vi "Check Scan Error.vi"(8 "error in (no error)":errorcluster {"code" format="%x"}, 10 "Response Input":string, 11 "VISA resource name":refnum<visa-resource-name>) -> (0 "error out":errorcluster {"code" format="%x"}, 2 "Response Output":string, 3 "VISA resource name out":refnum<visa-resource-name>)   [LabVIEW 2023, in "Bronkhorst FLOW-BUS.lvlib"]
doc: "This VI checks if the response string after a write/read sequence contains a status message. If is does, the error or warning contained in the status message is output in the <b>error out</b> cluster. \n\nFor information about the structure of error messages, please refer to chapter 3.3.3 and 3.6 of document 9.17.027."
uses:
  Bronkhorst FLOW-BUS.lvlib
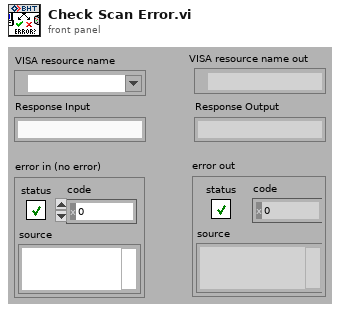
[diagram p1: front panel]
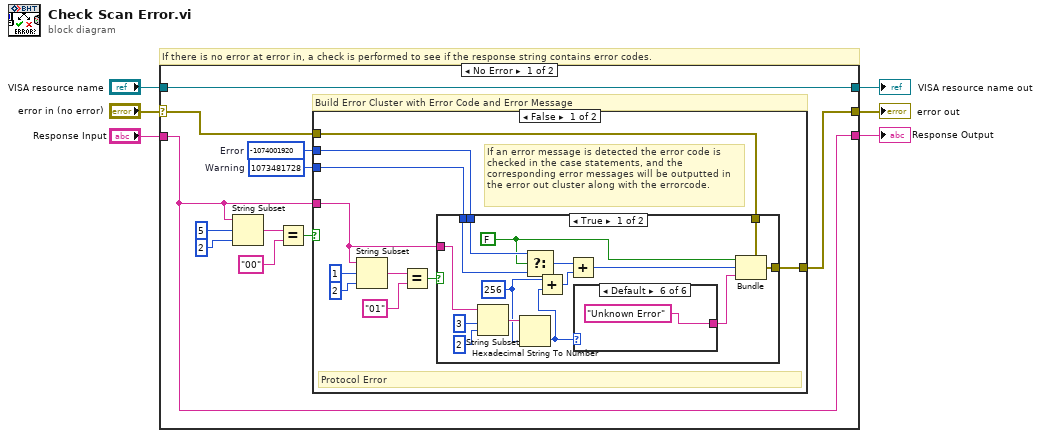
[diagram p0: block diagram]
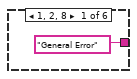
[diagram p2: hidden frame]
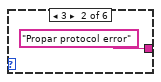
[diagram p3: hidden frame]
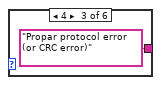
[diagram p4: hidden frame]
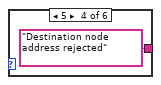
[diagram p5: hidden frame]
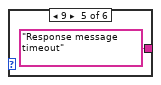
[diagram p6: hidden frame]
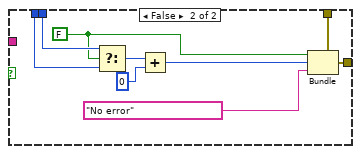
[diagram p7: hidden frame]
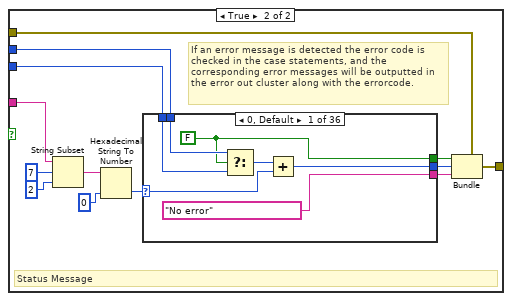
[diagram p8: hidden frame]
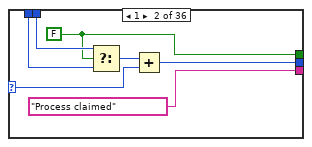
[diagram p9: hidden frame]
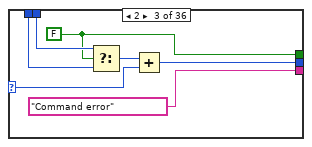
[diagram p10: hidden frame]
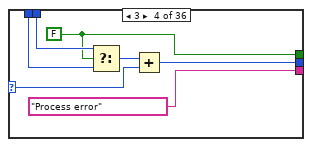
[diagram p11: hidden frame]
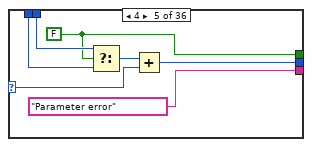
[diagram p12: hidden frame]
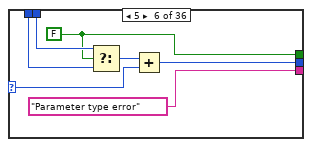
[diagram p13: hidden frame]
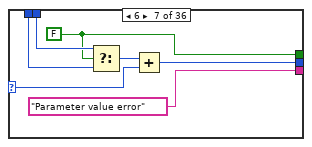
[diagram p14: hidden frame]
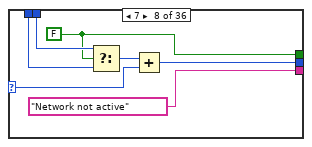
[diagram p15: hidden frame]
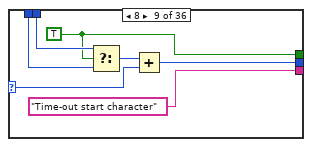
[diagram p16: hidden frame]
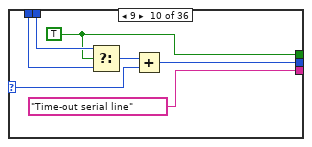
[diagram p17: hidden frame]
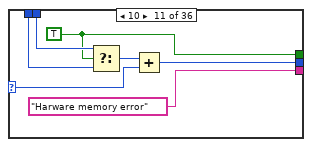
[diagram p18: hidden frame]
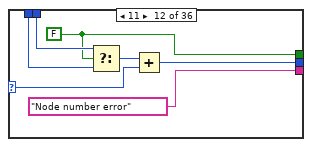
[diagram p19: hidden frame]
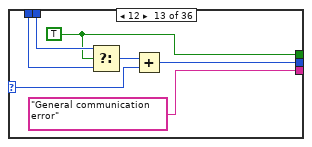
[diagram p20: hidden frame]
diagram:
  # "If there is no error at error in, a check is performed to see if the response string contains error codes."
  n1 = case shown="No Error" "error in (no error)" {
    selector: "error in (no error)" -> [w13 w325]
    tunnel: [w12 w325] -> w6
    tunnel: "Response Input" -> [w7 w323]
    tunnel: "VISA resource name" -> [w11 w324]
    tunnel: [w11 w324] -> w2
    tunnel: [w7 w323] -> w1
    frame No Error {
      w8 = 1073481728  # Warning
      w9 = -1074001920  # Error
      # "Build Error Cluster with Error Code and Error Message"
      n2 = String Subset(string=w7, offset (0)=u32 5 ("byte count (0)"), length (rest)=u32 2 ("byte count (0)")) -> (substring=w15:string)
      n3 = Equal?(x=w15, y="00" ("write buffer (\"\")")) -> (x = y?=w10:bool)
      n4 = case shown="False" w10 {
        tunnel: w7 -> [w20 w70]
        tunnel: w13 -> [w21 w66]
        tunnel: [w22 w65] -> w12
        tunnel: w9 -> [w19 w59]
        tunnel: w8 -> [w18 w58]
        frame False {
          # "Protocol Error"
          # "If an error message is detected the error code is checked in the case statements, and the corresponding error messages will be outputted in the error out cluster along with the errorcode."
          n5 = String Subset(string=w20, offset (0)=u32 1 ("byte count (0)"), length (rest)=u32 2 ("byte count (0)")) -> (substring=w23:string)
          n6 = Equal?(x=w23, y="01" ("write buffer (\"\")")) -> (x = y?=w26:bool)
          n7 = case shown="True" w26 {
            tunnel: w18 -> [w34 w55]
            tunnel: w19 -> [w35 w56]
            tunnel: w20 -> [w33 _]
            tunnel: [w32 w54] -> w22
            tunnel: w21 -> [w29 w52]
            frame True {
              w37 = 256 ("byte count (0)")
              w28 = FALSE
              n8 = String Subset(string=w33, offset (0)=u32 3 ("byte count (0)"), length (rest)=u32 2 ("byte count (0)")) -> (substring=w38:string)
              n9 = Hexadecimal String To Number(string=w38, default (0uL)=w37) -> (number=w36:i32)  [unwired: 1 in, 1 out]
              n10 = Select(t=w35, s=w28, f=w34) -> (s? t:f=w42:i32)
              n11 = Add(x=w37, y=w36) -> (x+y=w39:i32)
              n12 = Add(x=w42, y=w39) -> (x+y=w30:i32)
              n13 = case shown="Default" w36 {
                tunnel: ["General Error" "Propar protocol error" "Propar protocol error (or CRC error)" "Destination node address rejected" "Response message timeout" "Unknown Error"] -> w31
                frame 1, 2, 8 {
                }
                frame 3 {
                }
                frame 4 {
                }
                frame 5 {
                }
                frame 9 {
                }
                frame Default {
                }
              }
              n14 = Bundle(cluster=w29, "status"=w28, "code"=w30, "source"=w31) -> (w32:errorcluster)
            }
            frame False {
              w50 = FALSE
              n15 = Select(t=w56, s=w50, f=w55) -> (s? t:f=w57:i32)
              n16 = Add(x=w57, y=0) -> (x+y=w53:i32)
              n17 = Bundle(cluster=w52, "status"=w50, "code"=w53, "source"="No error") -> (w54:errorcluster)
            }
          }
        }
        frame True {
          # "Status Message"
          # "If an error message is detected the error code is checked in the case statements, and the corresponding error messages will be outputted in the error out cluster along with the errorcode."
          n18 = String Subset(string=w70, offset (0)=u32 7 ("byte count (0)"), length (rest)=u32 2 ("byte count (0)")) -> (substring=w67:string)
          n19 = Hexadecimal String To Number(string=w67, default (0uL)=0 ("I32")) -> (number=w63:i32)  [unwired: 1 in, 1 out]
          n20 = case shown="0, Default" w63 {
            selector: w63 -> [w73 w80 w87 w94 w101 w108 w115 w122 w129 w136 w143 w150 w157 w164 w171 w178 w185 w192 w199 w206 w213 w220 w227 w234 w241 w248 w255 w262 w269 w276 w283 w290 w297 w304 w311 w318]
            tunnel: w58 -> [w76 w83 w90 w97 w104 w111 w118 w125 w132 w139 w146 w153 w160 w167 w174 w181 w188 w195 w202 w209 w216 w223 w230 w237 w244 w251 w258 w265 w272 w279 w286 w293 w300 w307 w314 w321]
            tunnel: w59 -> [w75 w82 w89 w96 w103 w110 w117 w124 w131 w138 w145 w152 w159 w166 w173 w180 w187 w194 w201 w208 w215 w222 w229 w236 w243 w250 w257 w264 w271 w278 w285 w292 w299 w306 w313 w320]
            tunnel: [w74 w81 w88 w95 w102 w109 w116 w123 w130 w137 w144 w151 w158 w165 w172 w179 w186 w193 w200 w207 w214 w221 w228 w235 w242 w249 w256 w263 w270 w277 w284 w291 w298 w305 w312 w319] -> w60
            tunnel: ["No error" "Process claimed" "Command error" "Process error" "Parameter error" "Parameter type error" "Parameter value error" "Network not active" "Time-out start character" "Time-out serial line" "Harware memory error" "Node number error" "General communication error" "Read only parameter" "Error PC-communication" "No RS232 connection" "PC out of memory" "Write only parameter" "System configuration unknown" "No free node address" "Wrong interface type" "Error serial port connection" "Error opening communication" "Communication error" "Error interface bus master" "Timeout answer" "No start character" "Error first digit" "Buffer overflow in host" "Buffer overflow" "No answer found" "Error closing communication" "Synchronisation error" "Send error" "Protocol error" "Buffer overflow in module"] -> w62
            tunnel: [w71 w78 w85 w92 w99 w106 w113 w120 w127 w134 w141 w148 w155 w162 w169 w176 w183 w190 w197 w204 w211 w218 w225 w232 w239 w246 w253 w260 w267 w274 w281 w288 w295 w302 w309 w316] -> w61
            frame 0, Default {
              w74 = FALSE
              n21 = Select(t=w75, s=w74, f=w76) -> (s? t:f=w77:i32)
              n22 = Add(x=w77, y=w73) -> (x+y=w71:i32)
            }
            frame 1 {
              w81 = FALSE
              n23 = Select(t=w82, s=w81, f=w83) -> (s? t:f=w84:i32)
              n24 = Add(x=w84, y=w80) -> (x+y=w78:i32)
            }
            frame 2 {
              w88 = FALSE
              n25 = Select(t=w89, s=w88, f=w90) -> (s? t:f=w91:i32)
              n26 = Add(x=w91, y=w87) -> (x+y=w85:i32)
            }
            frame 3 {
              w95 = FALSE
              n27 = Select(t=w96, s=w95, f=w97) -> (s? t:f=w98:i32)
              n28 = Add(x=w98, y=w94) -> (x+y=w92:i32)
            }
            frame 4 {
              w102 = FALSE
              n29 = Select(t=w103, s=w102, f=w104) -> (s? t:f=w105:i32)
              n30 = Add(x=w105, y=w101) -> (x+y=w99:i32)
            }
            frame 5 {
              w109 = FALSE
              n31 = Select(t=w110, s=w109, f=w111) -> (s? t:f=w112:i32)
              n32 = Add(x=w112, y=w108) -> (x+y=w106:i32)
            }
            frame 6 {
              w116 = FALSE
              n33 = Select(t=w117, s=w116, f=w118) -> (s? t:f=w119:i32)
              n34 = Add(x=w119, y=w115) -> (x+y=w113:i32)
            }
            frame 7 {
              w123 = FALSE
              n35 = Select(t=w124, s=w123, f=w125) -> (s? t:f=w126:i32)
              n36 = Add(x=w126, y=w122) -> (x+y=w120:i32)
            }
            frame 8 {
              w130 = TRUE
              n37 = Select(t=w131, s=w130, f=w132) -> (s? t:f=w133:i32)
              n38 = Add(x=w133, y=w129) -> (x+y=w127:i32)
            }
            frame 9 {
              w137 = TRUE
              n39 = Select(t=w138, s=w137, f=w139) -> (s? t:f=w140:i32)
              n40 = Add(x=w140, y=w136) -> (x+y=w134:i32)
            }
            frame 10 {
              w144 = TRUE
              n41 = Select(t=w145, s=w144, f=w146) -> (s? t:f=w147:i32)
              n42 = Add(x=w147, y=w143) -> (x+y=w141:i32)
            }
            frame 11 {
              w151 = FALSE
              n43 = Select(t=w152, s=w151, f=w153) -> (s? t:f=w154:i32)
              n44 = Add(x=w154, y=w150) -> (x+y=w148:i32)
            }
            frame 12 {
              w158 = TRUE
              n45 = Select(t=w159, s=w158, f=w160) -> (s? t:f=w161:i32)
              n46 = Add(x=w161, y=w157) -> (x+y=w155:i32)
            }
            frame 13 {
              w165 = FALSE
              n47 = Select(t=w166, s=w165, f=w167) -> (s? t:f=w168:i32)
              n48 = Add(x=w168, y=w164) -> (x+y=w162:i32)
            }
            frame 14 {
              w172 = TRUE
              n49 = Select(t=w173, s=w172, f=w174) -> (s? t:f=w175:i32)
              n50 = Add(x=w175, y=w171) -> (x+y=w169:i32)
            }
            frame 15 {
              w179 = TRUE
              n51 = Select(t=w180, s=w179, f=w181) -> (s? t:f=w182:i32)
              n52 = Add(x=w182, y=w178) -> (x+y=w176:i32)
            }
            frame 16 {
              w186 = TRUE
              n53 = Select(t=w187, s=w186, f=w188) -> (s? t:f=w189:i32)
              n54 = Add(x=w189, y=w185) -> (x+y=w183:i32)
            }
            frame 17 {
              w193 = FALSE
              n55 = Select(t=w194, s=w193, f=w195) -> (s? t:f=w196:i32)
              n56 = Add(x=w196, y=w192) -> (x+y=w190:i32)
            }
            frame 18 {
              w200 = TRUE
              n57 = Select(t=w201, s=w200, f=w202) -> (s? t:f=w203:i32)
              n58 = Add(x=w203, y=w199) -> (x+y=w197:i32)
            }
            frame 19 {
              w207 = TRUE
              n59 = Select(t=w208, s=w207, f=w209) -> (s? t:f=w210:i32)
              n60 = Add(x=w210, y=w206) -> (x+y=w204:i32)
            }
            frame 20 {
              w214 = TRUE
              n61 = Select(t=w215, s=w214, f=w216) -> (s? t:f=w217:i32)
              n62 = Add(x=w217, y=w213) -> (x+y=w211:i32)
            }
            frame 21 {
              w221 = TRUE
              n63 = Select(t=w222, s=w221, f=w223) -> (s? t:f=w224:i32)
              n64 = Add(x=w224, y=w220) -> (x+y=w218:i32)
            }
            frame 22 {
              w228 = TRUE
              n65 = Select(t=w229, s=w228, f=w230) -> (s? t:f=w231:i32)
              n66 = Add(x=w231, y=w227) -> (x+y=w225:i32)
            }
            frame 23 {
              w235 = TRUE
              n67 = Select(t=w236, s=w235, f=w237) -> (s? t:f=w238:i32)
              n68 = Add(x=w238, y=w234) -> (x+y=w232:i32)
            }
            frame 24 {
              w242 = TRUE
              n69 = Select(t=w243, s=w242, f=w244) -> (s? t:f=w245:i32)
              n70 = Add(x=w245, y=w241) -> (x+y=w239:i32)
            }
            frame 25 {
              w249 = TRUE
              n71 = Select(t=w250, s=w249, f=w251) -> (s? t:f=w252:i32)
              n72 = Add(x=w252, y=w248) -> (x+y=w246:i32)
            }
            frame 26 {
              w256 = TRUE
              n73 = Select(t=w257, s=w256, f=w258) -> (s? t:f=w259:i32)
              n74 = Add(x=w259, y=w255) -> (x+y=w253:i32)
            }
            frame 27 {
              w263 = TRUE
              n75 = Select(t=w264, s=w263, f=w265) -> (s? t:f=w266:i32)
              n76 = Add(x=w266, y=w262) -> (x+y=w260:i32)
            }
            frame 28 {
              w270 = TRUE
              n77 = Select(t=w271, s=w270, f=w272) -> (s? t:f=w273:i32)
              n78 = Add(x=w273, y=w269) -> (x+y=w267:i32)
            }
            frame 29 {
              w277 = TRUE
              n79 = Select(t=w278, s=w277, f=w279) -> (s? t:f=w280:i32)
              n80 = Add(x=w280, y=w276) -> (x+y=w274:i32)
            }
            frame 30 {
              w284 = FALSE
              n81 = Select(t=w285, s=w284, f=w286) -> (s? t:f=w287:i32)
              n82 = Add(x=w287, y=w283) -> (x+y=w281:i32)
            }
            frame 31 {
              w291 = TRUE
              n83 = Select(t=w292, s=w291, f=w293) -> (s? t:f=w294:i32)
              n84 = Add(x=w294, y=w290) -> (x+y=w288:i32)
            }
            frame 32 {
              w298 = TRUE
              n85 = Select(t=w299, s=w298, f=w300) -> (s? t:f=w301:i32)
              n86 = Add(x=w301, y=w297) -> (x+y=w295:i32)
            }
            frame 33 {
              w305 = FALSE
              n87 = Select(t=w306, s=w305, f=w307) -> (s? t:f=w308:i32)
              n88 = Add(x=w308, y=w304) -> (x+y=w302:i32)
            }
            frame 34 {
              w312 = TRUE
              n89 = Select(t=w313, s=w312, f=w314) -> (s? t:f=w315:i32)
              n90 = Add(x=w315, y=w311) -> (x+y=w309:i32)
            }
            frame 35 {
              w319 = TRUE
              n91 = Select(t=w320, s=w319, f=w321) -> (s? t:f=w322:i32)
              n92 = Add(x=w322, y=w318) -> (x+y=w316:i32)
            }
          }
          n93 = Bundle(cluster=w66, "status"=w60, "code"=w61, "source"=w62) -> (w65:errorcluster)
        }
      }
    }
    frame Error {
    }
  }
  "VISA resource name out" <- w2
  "error out" <- w6
  "Response Output" <- w1
